vi "Drive Controller.vi"(8 "error in":errorcluster) -> ()   [LabVIEW 2019]
doc: "This VI executes continuously carrying out the current operation and responding to updates or new operation requests. It will often contain the timing or control code that is difficult to place directly in TeleOp. This VI generally opens all sensors and motors and isolates the rest of the robot code from knowing implementation details of how the operations are carried out."
uses:
  <vilib>/Rock Robotics/WPI/Framework/Completion Status.ctl
  Drive Setpoints.ctl
  Drive Operations.ctl
  Support Code/Single Cmd Info.ctl
  <vilib>/picture/picture.llb/imagedata.ctl
  Support Code/types/Limits.ctl
  <vilib>/Rock Robotics/WPI/ThirdParty/REV Robotics/SPARK MAX/Typedef/Spark MAX Control Type.ctl
panel:
  out "Left Setpoints":T1(graph)
  in  "Interactive Values":T2 {"Path stuff"."Limits"."Limits"."StoopidFast (fps)" min=0.0; "Path stuff"."Limits"."Limits"."Jerk (fps^3)" min=0.0 step=1.0; "Path stuff"."Limits"."Limits"."Accel (fps^2)" min=0.0; "Path stuff"."Limits"."Limits"."Velocity (fps)" min=0.0}
  in  "Buttons":cluster{"Execute Cmd":bool, "Abort Cmd":bool}
  out "Command Timing":cluster{"Start Time (ms)":u32, "Iterations":i32}
  out "Status":T7
  out "Right Setpoints":T1(graph)
  out "Current\nCmd":string
  # "Tip: The graph shows the motor setpoints. It may also be helpful to observe inputs and sensor values.\nYou may also want to display tuning or debugging controls."
  # "Interactive Command: You may fill in the settings for a command\nand schedule it with the Execute button. You can observe and abort\nany command while fine tuning the code for the controller."
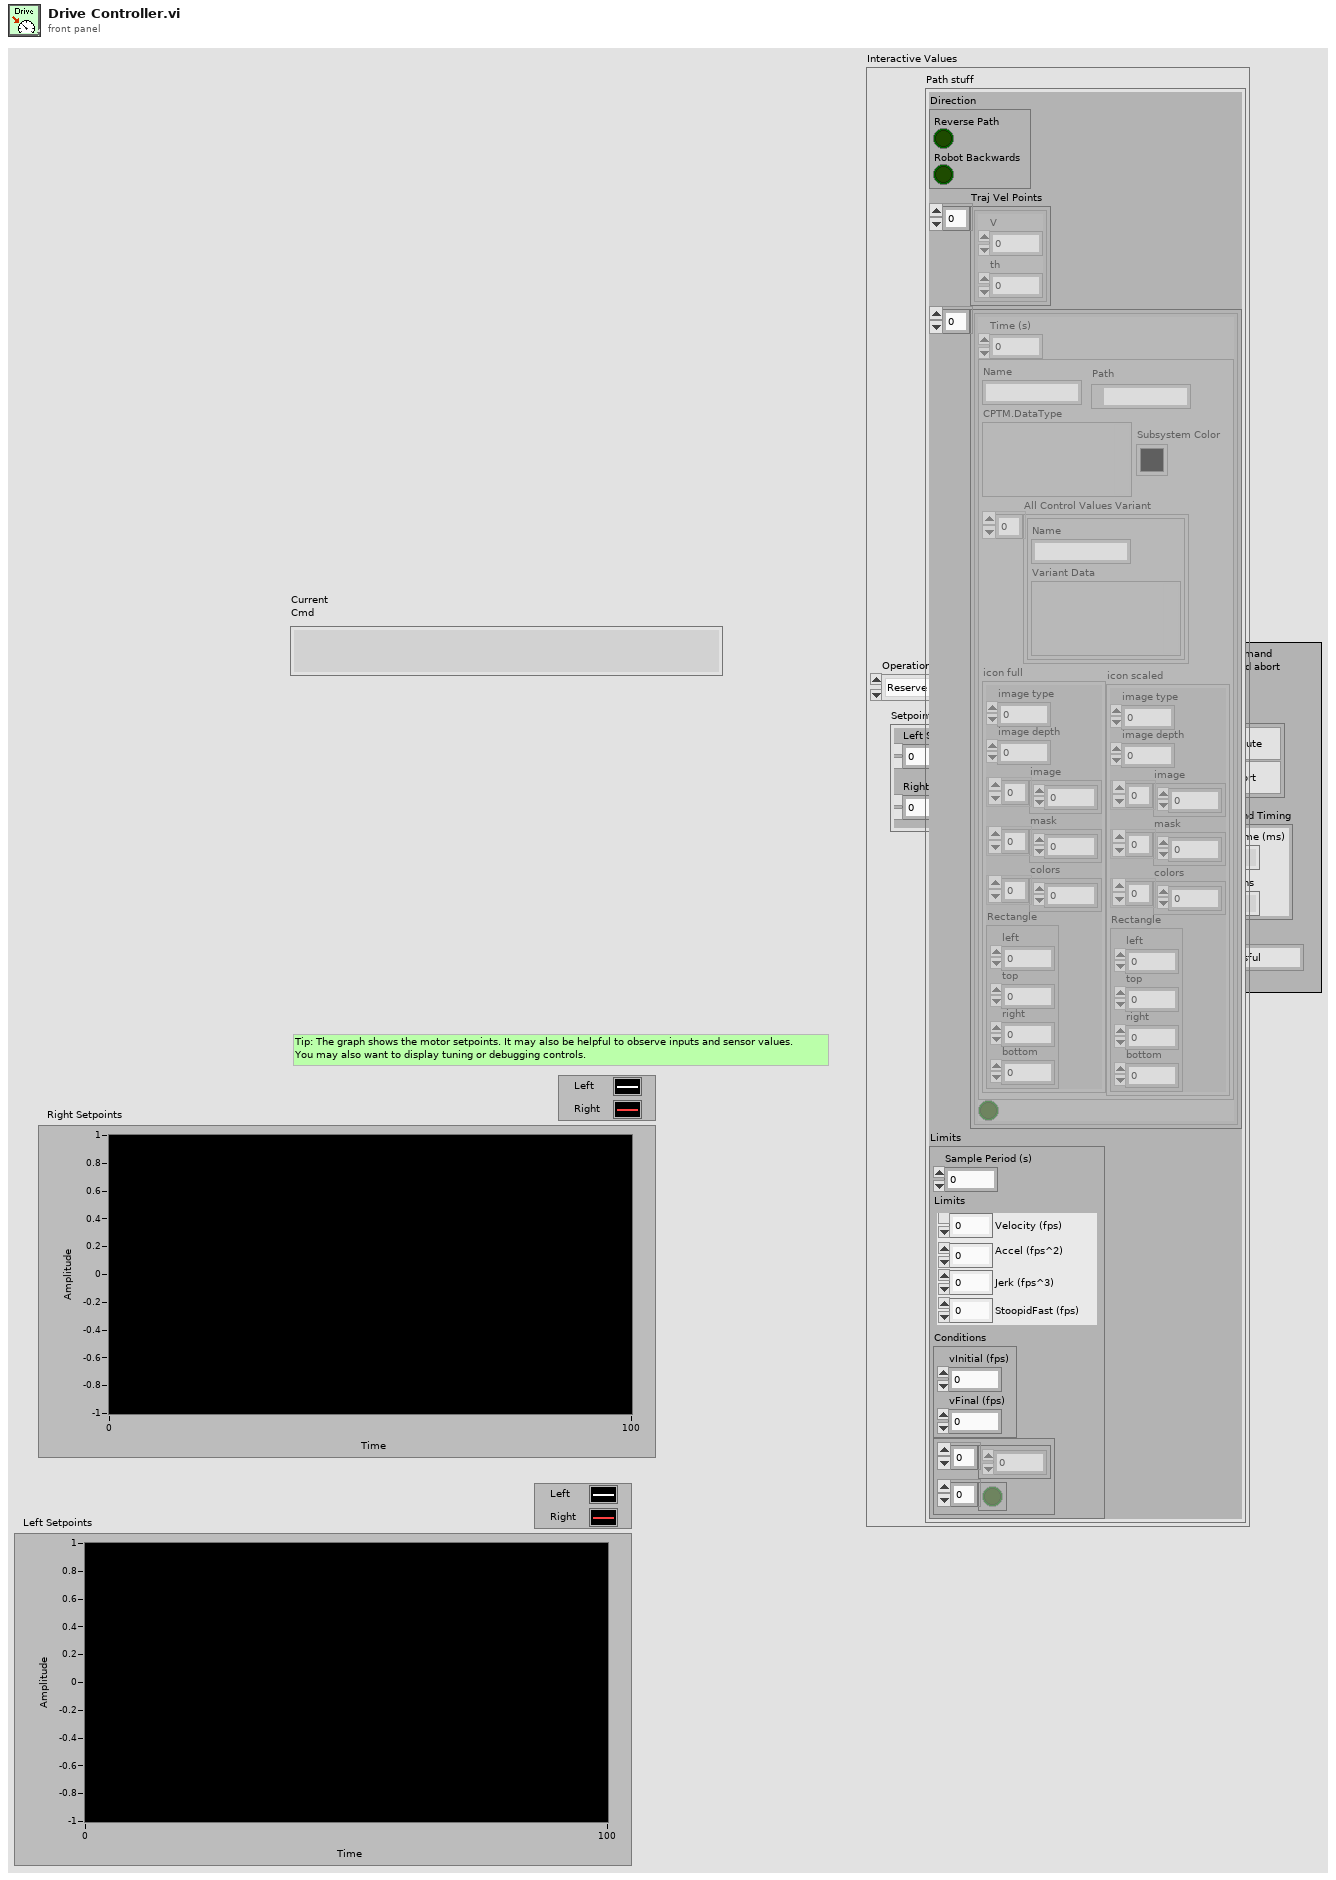
[diagram p1: front panel]
types:
  T1 = cluster{"Left Setpoint":dbl, "Right Setpoint":dbl}
  T2 = typedef "Drive Setpoints.ctl" = cluster{"Operation":T3, "Setpoints":cluster{"Left Setpoint":dbl, "Right Setpoint":dbl}, "Path stuff":cluster{"Direction":cluster{"Reverse Path":bool, "Robot Backwards":bool}, "Traj Vel Points":cluster{"V":dbl, "th":dbl}[], "Commands":cluster{"Time (s)":dbl, T4, bool}[], "Limits":cluster{"Sample Period (s)":dbl, "Limits":T6, "Conditions":cluster{"vInitial (fps)":dbl, "vFinal (fps)":dbl}, cluster{dbl[], bool[]}}}}
  T3 = typedef "Drive Operations.ctl" = enum16{"Reserve", "Read Current", "Immediate", "Play Path"}
  T4 = typedef "Single Cmd Info.ctl" = cluster{"Name":string, "CPTM.DataType":variant, "All Control Values Variant":cluster{"Name":string, "Variant Data":variant}[], "icon full":T5, "icon scaled":T5, "Path":path, "Subsystem Color":u32}
  T5 = typedef "imagedata.ctl" = cluster{"image type":i32, "image depth":i32, "image":u8[], "mask":u8[], "colors":u32[], "Rectangle":cluster{"left":i16, "top":i16, "right":i16, "bottom":i16}}
  T6 = typedef "Limits.ctl" = cluster{"Velocity (fps)":dbl, "Accel (fps^2)":dbl, "Jerk (fps^3)":dbl, "StoopidFast (fps)":dbl}
  T7 = typedef "Completion Status.ctl" = enum16{"Successful", "Aborted", "Incomplete"}
  T8 = cluster{"P Gain":dbl, "I Gain":dbl, "D Gain":dbl, "F Gain":dbl, "I Zone":dbl, "Min Output":dbl, "Max Output":dbl}
  T9 = typedef "Command Status Info.ctl" = cluster{"Name":string, "Status":T7, "notifier out":T10}
  T10 = typedef "Completion Notifier.ctl" = refnum<notifier>
  T11 = cluster{"SubSystem Data":T2, cluster{"Start Time (ms)":u32, "Iterations":i32}, cluster{"Command Info":T9, "Description":string, "Default Command":T2, "queue out":refnum<queue>, "Subsystem Name":string}}
  T12 = typedef "WPI_MotorControlDeviceRef.ctl" = cluster{"DeviceStatus":errorcluster, "Type":T13, "PWM":cluster{"PWM Channel":T14, "DeadBand":T15}, "CAN":cluster{"Device Number":u8, "SetOutput VI Ref":variant, "GetOutput VI Ref":variant, "Enable VI Ref":variant, "Disable VI Ref":variant, "Data":variant}, "Invert":bool, "DIO PWM":cluster{"PWM \"Enable\" Channel":T14, "DIOChannel":T16, "PWM Rate":dbl}}
  T13 = typedef "WPI_MotorControlType.ctl" = enum16{"PWM", "CAN", "DIO PWM"}
  T14 = typedef "FPGA_DIOPWMChannel.ctl" = enum8{"PWM 0", "PWM 1", "PWM 2", "PWM 3", "PWM 4", "PWM 5", "PWM 6", "PWM 7", "PWM 8", "PWM 9", "PWM MXP 0", "PWM MXP 1", "PWM MXP 2", "PWM MXP 3", "PWM MXP 4", "PWM MXP 5", "PWM MXP 6", "PWM MXP 7", "PWM MXP 8", "PWM MXP 9", "Invalid"}
  T15 = typedef "WPI_PWMDeadband.ctl" = cluster{"Name":string, "maxPositivePwm":i32, "minPositivePwm":i32, "centerPwm":i32, "maxNegativePwm":i32, "minNegativePwm":i32, "angularRange":u16}
  T16 = typedef "FPGA_DIOChannel.ctl" = enum8{"DIO 0", "DIO 1", "DIO 2", "DIO 3", "DIO 4", "DIO 5", "DIO 6", "DIO 7", "DIO 8", "DIO 9", "DIO MXP 0", "DIO MXP 1", "DIO MXP 2", "DIO MXP 3", "DIO MXP 4", "DIO MXP 5", "DIO MXP 6", "DIO MXP 7", "DIO MXP 8", "DIO MXP 9", "DIO MXP 10", "DIO MXP 11", "DIO MXP 12", "DIO MXP 13", "DIO MXP 14", "DIO MXP 15", "SPI Port CS1", "SPI Port CS2", "SPI Port CS3", "SPI Port MISO", "SPI Port MOSI", "Invalid"}
  T17 = typedef "ADIS16470 Device Reference.ctl" = cluster{"DevStatus":errorcluster, "Hardware Config":T18, "Calibration Complete":refnum<notifier>, "Status FIFO":refnum<k33>, "Last Value Reference":refnum<data-value>, "Sychronous Process VI":T21, "Cmd FIFO":refnum<k33>, "Source":T22, "Data FIFO":refnum<k33>, "Calibration Time":T26}
  T18 = typedef "ADIS16470 Hardware Configuration.ctl" = cluster{"SPI Clock Rate (Hz)":dbl, "IMU SPI Mode (3)":T19, "IMU Reset Pin":T16, "IMU SPI Bus":T20, "IMU Data Ready Pin":T16, "Stall Config":cluster{"Pow2BytesPerRead":u8, "StallTicks":u16, "CsToSclkTicks":u8}}
  T19 = typedef "WPI_SPIMode.ctl" = enum16{"Mode 0 (Clk Idle Low,Sample on Leading)", "Mode 1 (Clk Idle Low,Sample on Trailing)", "Mode 2 (Clk Idle High,Sample on Leading)", "Mode 3 (Clk Idle High,Sample on Trailing)"}
  T20 = typedef "spi_bus.ctl" = enum16{"SPI On-Board, CS0", "SPI On-Board, CS1", "SPI On-Board, CS2", "SPI On-Board, CS3", "SPI MXP", "Invalid"}
  T21 = typedef "ADIS16470 Process.ctl" = refnum<vi>
  T22 = typedef "FPGA_CounterEncoderSourceConvertionLVSourceType.ctl" = cluster{"DevStatus":errorcluster, "AnalogTriggerMode?":bool, "DigitalMode":cluster{"DIO Channel":T23}, "AnalogTriggerMode":cluster{"AnalogTriggerIndex":T24, "OutputType":T25}}
  T23 = typedef "FPGA_DIODigitalSourceChannel.ctl" = enum8{"DIO 0", "DIO 1", "DIO 2", "DIO 3", "DIO 4", "DIO 5", "DIO 6", "DIO 7", "DIO 8", "DIO 9", "DIO MXP 0", "DIO MXP 1", "DIO MXP 2", "DIO MXP 3", "DIO MXP 4", "DIO MXP 5", "DIO MXP 6", "DIO MXP 7", "DIO MXP 8", "DIO MXP 9", "DIO MXP 10", "DIO MXP 11", "DIO MXP 12", "DIO MXP 13", "DIO MXP 14", "DIO MXP 15", "SPI Port CS1", "SPI Port CS2", "SPI Port CS3", "SPI Port MISO", "SPI Port MOSI", "Disabled"}
  T24 = typedef "FPGA_AnalogTriggerIndex.ctl" = enum8{"Trig 0", "Trig 1", "Trig 2", "Trig 3", "Trig 4", "Trig 5", "Trig 6", "Trig 7", "Invalid"}
  T25 = typedef "FPGA_AnalogTriggerOutType.ctl" = enum16{"InWindow", "TriggerState", "Rising", "Falling"}
  T26 = typedef "ADIS16470 Calibration Time.ctl" = enum16{"32ms", "64ms", "128ms", "256ms", "512ms", "1s", "2s", "4s", "8s", "16s", "32s", "64s"}
  T27 = typedef "Spark MAX Control Type.ctl" = enum16{"Percent VBus", "Voltage", "Velocity", "Position", "Smart Motion", "Current", "Smart Velocity"}
  T28 = cluster{"Direction":cluster{"Reverse Path":bool, "Robot Backwards":bool}, "Traj Vel Points":cluster{"V":dbl, "th":dbl}[], "Commands":cluster{"Time (s)":dbl, T4, bool}[], "Limits":cluster{"Sample Period (s)":dbl, "Limits":T6, "Conditions":cluster{"vInitial (fps)":dbl, "vFinal (fps)":dbl}, cluster{dbl[], bool[]}}}
  T29 = typedef "ADIS16470 Data.ctl" = cluster{"XAngle":dbl, "YAngle":dbl, "ZAngle":dbl}
  T30 = cluster{"SubSystem Data":T2, cluster{"Start Time (ms)":u32, "Iterations":i32}, "Default Command Arguments":cluster{"Command Info":T9, "Description":string, "Default Command":T2, "queue out":refnum<queue>, "Subsystem Name":string}}
  T31 = cluster{"Don't move motors while reserved":dbl, "Applied Output":dbl}
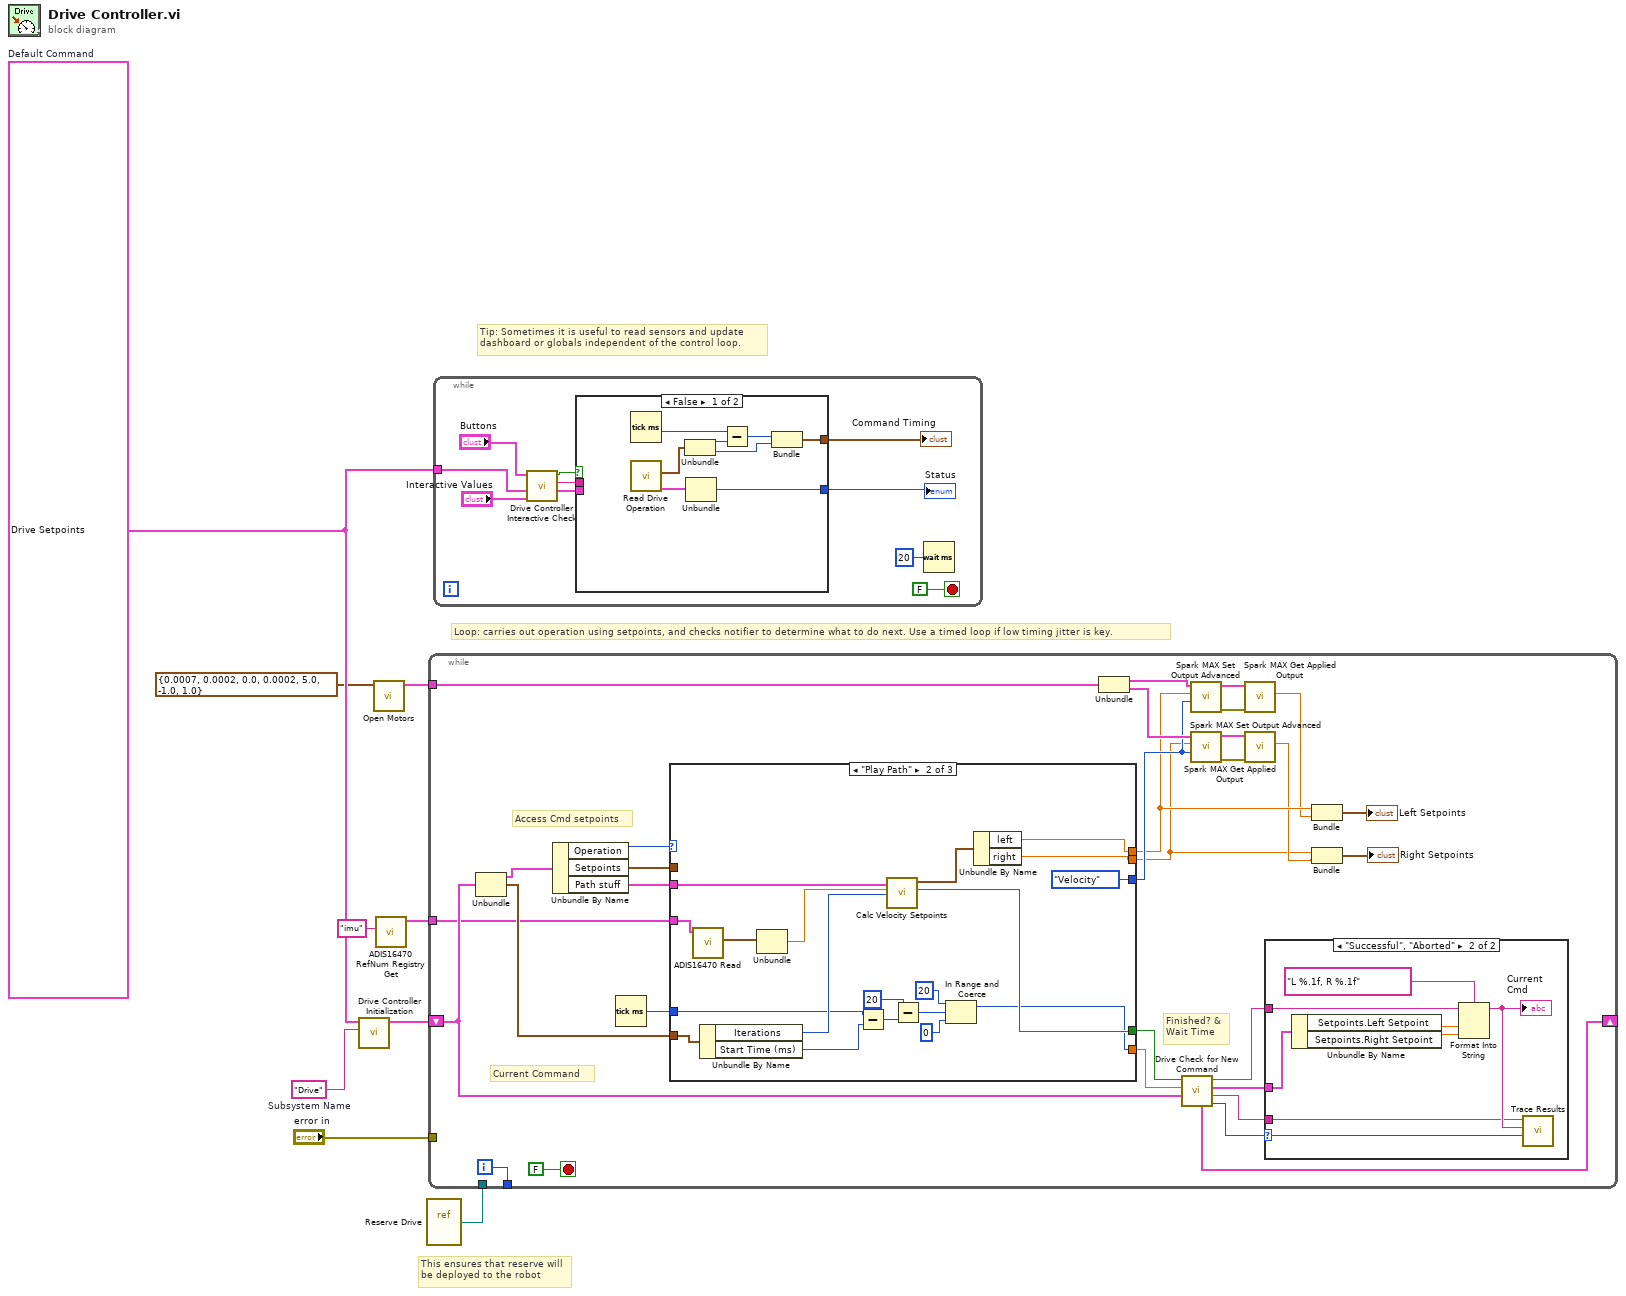
[diagram p0: block diagram]
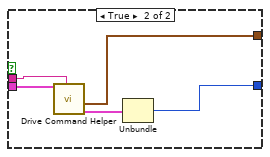
[diagram p2: hidden frame]
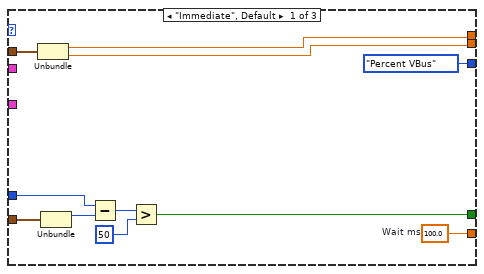
[diagram p4: hidden frame]
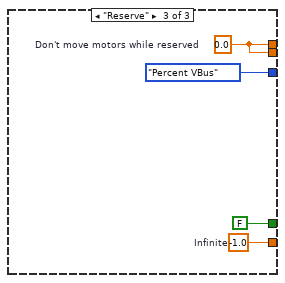
[diagram p5: hidden frame]
diagram:
  w5 = T2 {"Operation"=enum."Reserve", "Setpoints"={"Left Setpoint"=0.0, "Right Setpoint"=0.0}, "Path stuff"={"Direction"={"Reverse Path"=FALSE, "Robot Backwards"=FALSE}, "Traj Vel Points"=[], "Commands"=[], "Limits"={"Sample Period (s)"=0.0, "Limits"={"Velocity (fps)"=0.0, "Accel (fps^2)"=0.0, "Jerk (fps^3)"=0.0, "StoopidFast (fps)"=0.0}, "Conditions"={"vInitial (fps)"=0.0, "vFinal (fps)"=0.0}, {[], []}}}}  # Default Command
  w9 = "Drive"  # Subsystem Name
  # "This ensures that reserve will\nbe deployed to the robot"
  # "Tip: Sometimes it is useful to read sensors and update\ndashboard or globals independent of the control loop."
  # "Loop: carries out operation using setpoints, and checks notifier to determine what to do next. Use a timed loop if low timing jitter is key."
  n1 = call "Drive Controller Initialization.vi"("Subsystem Name"=w9, "Default Command"=w5) -> ("Current Command"=w7:T11)  [unwired: 9 in]
  n2 = call "Open Motors.vi"("PID Constants for Sparks"=T8 {"P Gain"=0.0007, "I Gain"=0.0002, "D Gain"=0.0, "F Gain"=0.0002, "I Zone"=5.0, "Min Output"=-1.0, "Max Output"=1.0}) -> ("motors"=w4:cluster{"left master":T12, "right master":T12})  [unwired: 9 in, 1 out]
  n3 = call "ADIS16470 RefNum Registry Get.vi"("refnum name"="imu") -> ("ADIS16470DevRef out"=w1:T17)  [unwired: 9 in, 1 out]
  n4 = vi-ref "Reserve Drive.vi"() -> (w6:refnum<vi>)
  n5 = while {
    shift-right: [w34] -> _
    shift-left: w7 -> [w27]
    tunnel: [w39] -> _
    tunnel: "error in" -> [_]
    tunnel: w6 -> [_]
    tunnel: w4 -> [w25]
    tunnel: w1 -> [w10]
    i -> [w39]
    stop <- FALSE stop-if-true
    # "Current Command"
    # "Access Cmd setpoints"
    # "Finished? &\nWait Time"
    n6 = Unbundle(w27) -> ("SubSystem Data"=w38:T2, w28:cluster{"Start Time (ms)":u32, "Iterations":i32})  [unwired: 1 out]
    n7 = Unbundle By Name(w38) -> ("Operation"=w37:T3, "Setpoints"=w26:T1, "Path stuff"=w11:T28)
    n8 = Tick Count (ms)() -> (millisecond timer value=w36:u32)
    n9 = case shown="\"Play Path\"" w37 {
      tunnel: [w59 w63 w82] -> w33
      tunnel: [w54 w74 FALSE ("ignore previous (F)")] -> w32
      tunnel: w28 -> [w53 w77 _]
      tunnel: [w50 w72 w80] -> w16
      tunnel: [w49 w71 w80] -> w12
      tunnel: w36 -> [w55 w69 _]
      tunnel: w26 -> [w52 _ _]
      tunnel: [Spark_MAX_Control_Type."Percent VBus" ("Control Mode") Spark_MAX_Control_Type."Velocity" ("Control Mode") Spark_MAX_Control_Type."Percent VBus" ("Control Mode")] -> w22
      tunnel: w11 -> [_ w75 _]
      tunnel: w10 -> [_ w62 _]
      frame "Immediate", Default {
        w59 = 100.0  # Wait ms
        n10 = Unbundle(w52) -> ("Left Setpoint"=w50:dbl, "Right Setpoint"=w49:dbl)
        n11 = Unbundle(w53) -> ("Start Time (ms)"=w56:u32)  [unwired: 1 out]
        n12 = Subtract(x=w55, y=w56) -> (x-y=w57:u32)
        n13 = Greater?(x=w57, y=u8 50 ("Left Motor")) -> (0:w54:bool)
      }
      frame "Play Path" {
        n14 = call "ADIS16470 Read.vi"("ADIS16470DevRef"=w62) -> ("ADIS16470 Value"=w61:T29)  [unwired: 7 in, 3 out]
        n15 = Unbundle By Name(w77) -> ("Iterations"=w76:i32, "Start Time (ms)"=w70:u32)
        n16 = Unbundle(w61) -> ("YAngle"=w60:dbl)  [unwired: 2 out]
        n17 = Subtract(x=w69, y=w70) -> (x-y=w68:u32)
        n18 = call "Calc Velocity Setpoints.vi"("Iterations"=w76, "Angle"=w60, "Path stuff"=w75) -> ("finished?"=w74:bool, "setpoints"=w73:cluster{"left":dbl, "right":dbl})  [unwired: 7 in]
        n19 = Subtract(x=u32 20, y=w68) -> (x-y=w66:u32)
        n20 = In Range and Coerce(upper limit=u32 20, x=w66, lower limit=u32 0) -> (coerced(x)=w63:u32)  [unwired: 1 out]
        n21 = Unbundle By Name(w73) -> ("left"=w72:dbl, "right"=w71:dbl)
      }
      frame "Reserve" {
        w80 = 0.0  # Don't move motors while reserved
        w82 = -1.0  # Infinite
      }
    }
    n22 = Unbundle(w25) -> ("left master"=w24:T12, "right master"=w23:T12)
    n23 = call "Drive Check for New Command.vi"("input cluster"=w27, "Wait time (ms)"=w33, "Finished?"=w32) -> ("Completion"=w35:T7, "Subsystem Name"=w29:string, "Current Command"=w30:T2, "Initial Trace String"=w31:string, "Next Command"=w34:T30)  [unwired: 4 in]
    n24 = call <vilib>:"Spark MAX Set Output Advanced.vi"("Control Mode"=w22, "Setpoint"=w16, "MotorControlDevRef"=w24) -> ("error out"=w21:errorcluster, "MotorControlDevRef"=w20:T12)  [unwired: 7 in]
    n25 = call <vilib>:"Spark MAX Set Output Advanced.vi"("Control Mode"=w22, "Setpoint"=w12, "MotorControlDevRef"=w23) -> ("error out"=w18:errorcluster, "MotorControlDevRef"=w19:T12)  [unwired: 7 in]
    n26 = call <vilib>:"Spark MAX Get Applied Output.vi"("error in (no error)"=w21, "MotorControlDevRef in"=w20) -> ("Applied Output"=w15:dbl)  [unwired: 6 in, 3 out]
    n27 = call <vilib>:"Spark MAX Get Applied Output.vi"("error in (no error)"=w18, "MotorControlDevRef in"=w19) -> ("Applied Output"=w14:dbl)  [unwired: 6 in, 3 out]
    n28 = case shown="\"Successful\", \"Aborted\"" w35 {
      selector: w35 -> [_ w48]
      tunnel: w31 -> [_ w43]
      tunnel: w30 -> [_ w44]
      tunnel: w29 -> [_ w41]
      frame "Incomplete", Default {
        # "Continuing current command"
      }
      frame "Successful", "Aborted" {
        # "Report and setup for next command"
        n29 = Unbundle By Name(w44) -> ("Setpoints.Left Setpoint"=w46:dbl, "Setpoints.Right Setpoint"=w47:dbl)
        n30 = Format Into String(format string="L %.1f, R %.1f", initial string=w43, w46, w47) -> (resulting string=w42:string)  [unwired: 1 in, 1 out]
        "Current\nCmd" <- w42
        n31 = call <vilib>:"Trace Results.vi"("Status of previous command"=w48, "Description"=w42, "Subsystem"=w41) -> ()  [unwired: 9 in]
      }
    }
    n32 = Bundle("Don't move motors while reserved"=w16, "Applied Output"=w15) -> (→"Left Setpoints":T31)  [unwired: 1 in]
    n33 = Bundle("Don't move motors while reserved"=w12, "Applied Output"=w14) -> (→"Right Setpoints":T31)  [unwired: 1 in]
  }
  n34 = while {
    tunnel: w5 -> [w85]
    stop <- FALSE stop-if-true
    n35 = call "Drive Controller Interactive Check.vi"("Interactive Command In"="Interactive Values", "Default Command"=w85, "Buttons"="Buttons") -> ("Interactive Command Out"=w87:T2, "Trace String"=w88:string, "Schedule"=w89:bool)  [unwired: 6 in]
    n36 = case shown="False" w89 {
      tunnel: [w97 w105] -> w90
      tunnel: [w93 w101] -> w83
      tunnel: w88 -> [_ w103]
      tunnel: w87 -> [_ w102]
      frame False {
        n37 = Tick Count (ms)() -> (millisecond timer value=w100:u32)
        n38 = call "Read Drive Operation.vi"() -> ("Command Info"=w95:T9, "Command Timing"=w94:cluster{"Start Time (ms)":u32, "Iterations":i32})  [unwired: 9 in, 1 out]
        n39 = Unbundle(w94) -> ("Start Time (ms)"=w98:u32, "Iterations"=w96:i32)
        n40 = Unbundle(w95) -> ("Status"=w97:T7)  [unwired: 2 out]
        n41 = Subtract(x=w100, y=w98) -> (x-y=w99:u32)
        n42 = Bundle(w99, "Iterations"=w96) -> (w93:cluster{u32, "Iterations":i32})  [unwired: 1 in]
      }
      frame True {
        n43 = call "Drive Command Helper.vi"("Description"=w103, "SubSystem Data"=w102) -> ("Command Info Out"=w104:T9, "Command Timing"=w101:cluster{"Start Time (ms)":u32, "Iterations":i32})  [unwired: 7 in, 1 out]
        n44 = Unbundle(w104) -> ("Status"=w105:T7)  [unwired: 2 out]
      }
    }
    "Status" <- w90
    "Command Timing" <- w83
    n45 = Wait (ms)(milliseconds to wait=u32 20) -> ()  [unwired: 1 out]
  }
